vi "多影像平均_二值化_抓邊 - 複製.vi"() -> ()   [LabVIEW 2015]
uses:
  <vilib>/vision/Measure.llb/Edge Options.ctl
  <vilib>/vision/Measure.llb/Edge Polarity.ctl
  <vilib>/userdefined/High Color/IMAQdx.ctl
  <vilib>/Utility/miscctls.llb/LVPositionTypeDef.ctl
  <vilib>/vision/NI_Vision_Development_Module.lvlib
  <vilib>/vision/driver/NI_Vision_Acquisition_Software.lvlib
  <resource>/objmgr/imaqdx.rc
panel:
  in  "載入影像":bool
  in  "拍攝影像":bool
  in  "影像數量":i32=4
  out "二值化影像陣列":T1[](array[plugin-control])
  out "全部影像Histograph":T2(graph)
  out "Image binary":T1(plugin-control)
  out "平均影像Histograph":T3(graph)
  out "Standard Deviation":sgl format="%#.2f"
  out "Mean":sgl format="%#.2f"
  out "影像陣列":T1[](array[plugin-control])
  in  "stop":bool
  in  "Horizontal Progress Bar":u8(slide) scale=0.0..255.0
  out "Image mean":T1(plugin-control)
  out "取像編號":i32
  out "取像視窗":T1(plugin-control)
  in  "Session In":T4="cam1"
  out "degrees":sgl
  in  "單點":bool
  in  "Edge Options":T5={"Edge Polarity"=0, "Kernel Size"=3, "Width"=3, "Minimum Edge Strength"=10.0, "Interpolation Type"=enum."Bilinear Fixed", "Data Processing Method"=enum."Average"} {"Edge Polarity" items=["All Edges", "Rising Edges", "Falling Edges"]; "Minimum Edge Strength" format="%.2f"; "Width" step=2; "Kernel Size" step=2}
  out "Gradient Information":dbl[][](graph)
  out "Line Segment":T7 {"Point 2"."Y" format="%.2f"; "Point 2"."X" format="%.2f"; "Point 1"."Y" format="%.2f"; "Point 1"."X" format="%.2f"}
  out "error out":errorcluster
  in  "Direction":T8(ring)
  in  "Process":u16(ring) items=["Get First Edge", "Get First + Last Edge", "Get All Edges", "Get Best Edge"]
  out "Line Profile":T9(graph)
  in  "Gap":i32=10
  out "Image":T1(plugin-control)
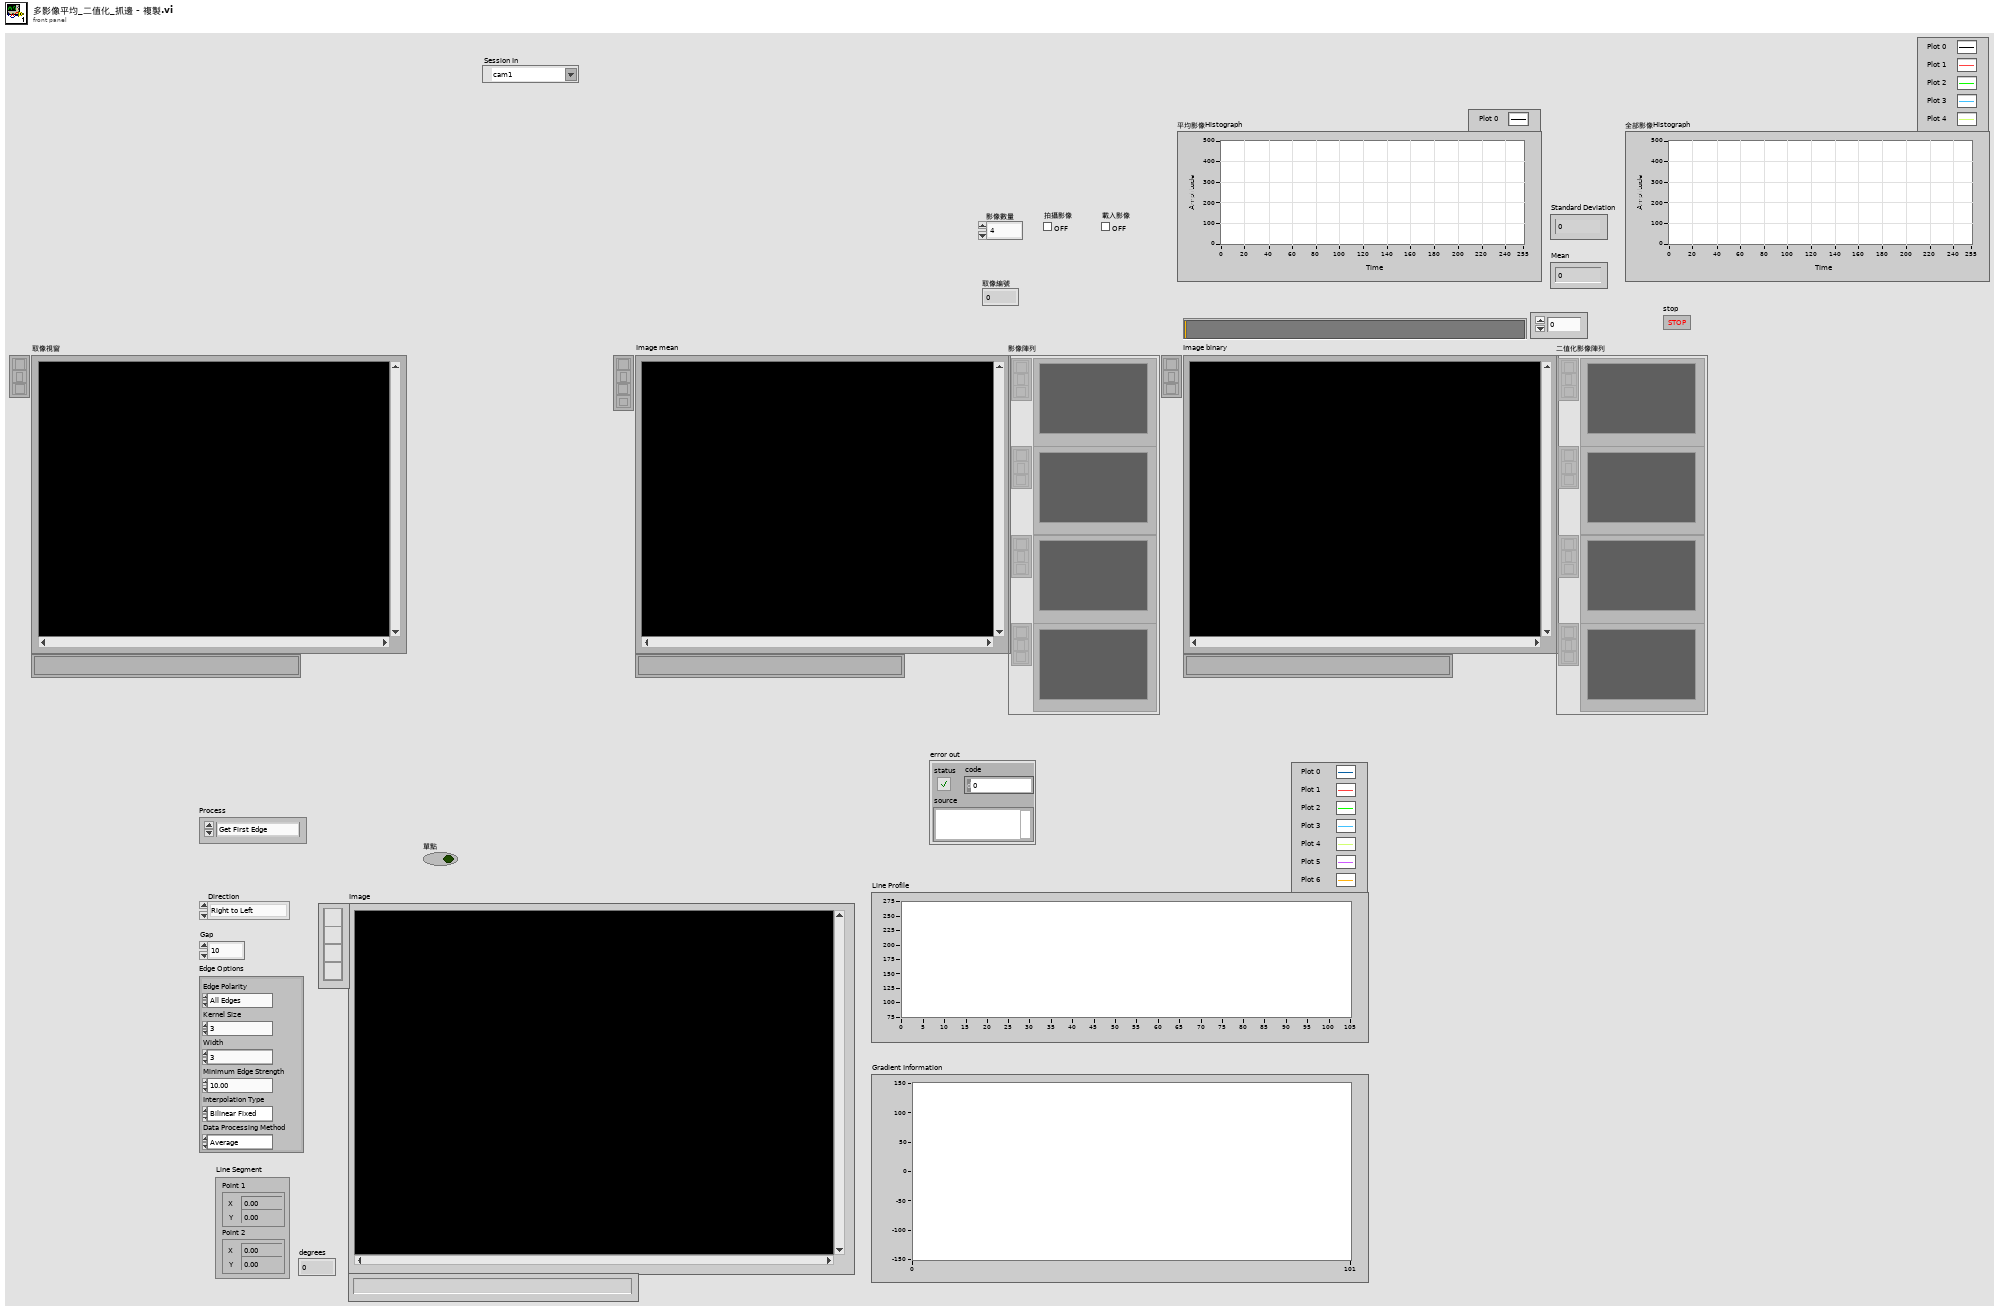
[diagram p1: front panel]
types:
  T1 = typedef "IMAQ Image.ctl" = refnum<image>
  T2 = cluster{"Starting Value":sgl, "Incremental Value":sgl, "Histogram":u32[]}[]
  T3 = cluster{"Starting Value":sgl, "Incremental Value":sgl, "Histogram":u32[]}
  T4 = typedef "IMAQdx.ctl" = refnum<k21>
  T5 = typedef "Edge Options.ctl" = cluster{"Edge Polarity":T6, "Kernel Size":u32, "Width":u32, "Minimum Edge Strength":sgl, "Interpolation Type":enum32{"Zero Order", "Bilinear", "Quadratic", "Cubic", "Bilinear Fixed"}, "Data Processing Method":enum32{"Average", "Median"}}
  T6 = typedef "Edge Polarity.ctl" = u32
  T7 = cluster{"Point 1":cluster{"X":sgl, "Y":sgl}, "Point 2":cluster{"X":sgl, "Y":sgl}}
  T8 = enum16{"Right to Left", "Left  to Right", "Up to Down", "Down to Up"}
  T9 = cluster{"x0":sgl, "dx":sgl, "Pixels Line":sgl[]}[]
  T10 = typedef "LVPositionTypeDef.ctl" = cluster{"Left":i32, "Top":i32}
  T11 = typedef "Image Type" = u32
  T12 = cluster{"Global Rectangle":i32[], "Contours":cluster{"Contour Type":u32, "ROI Type":u32, "Points":i32[]}[]}
  T13 = typedef "IMAQ Rectangle" = cluster{"Left":i32, "Top":i32, "Right":i32, "Bottom":i32, "Rotation":dbl}
  T14 = typedef "IMAQ Line" = cluster{"Start X":i32, "Start Y":i32, "End X":i32, "End Y":i32}
  T15 = typedef "IMAQ Point" = cluster{"X":sgl, "Y":sgl}
  T16 = typedef "ROI Descriptor" = cluster{"Global Rectangle":i32[], "Contours":cluster{"ID":enum32{"External", "Internal"}, "Type":u32, "Coordinates":i32[]}[]}
  T17 = typedef "Edge New.ctl" = cluster{"Location (Pixel)":cluster{"X":sgl, "Y":sgl}, "Location (Real-World)":cluster{"X":sgl, "Y":sgl}, "Distance (Pixel)":dbl, "Distance (Real-World)":dbl, "Strength":dbl, "Noise":dbl, "Rising?":bool}
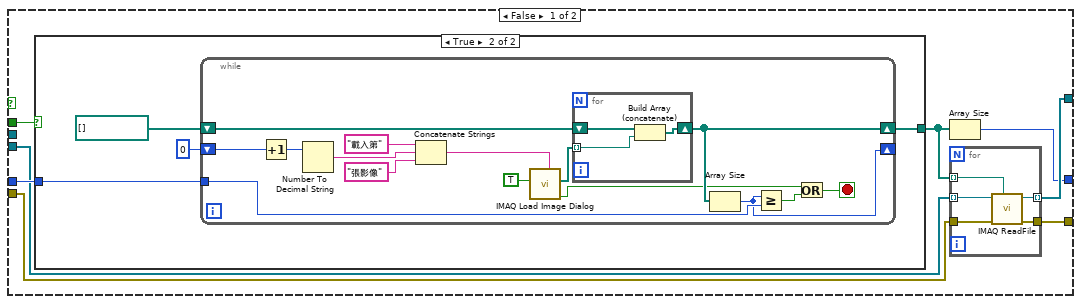
[diagram p2: hidden frame]
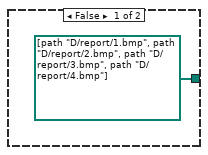
[diagram p3: hidden frame]
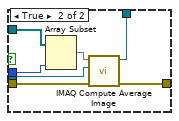
[diagram p4: hidden frame]
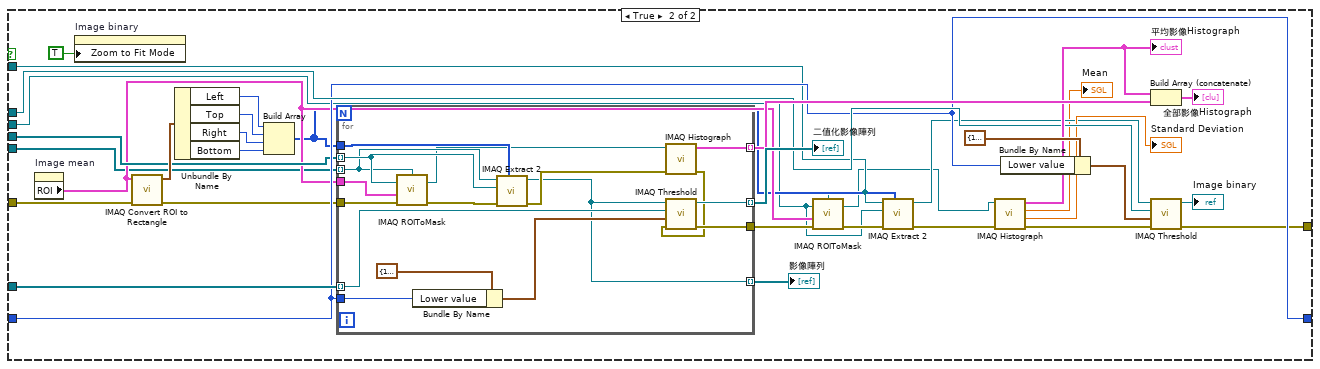
[diagram p5: hidden frame]
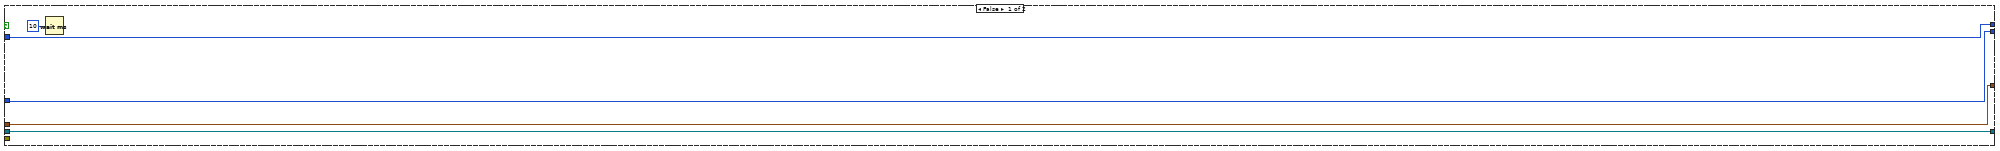
[diagram p6: hidden frame]
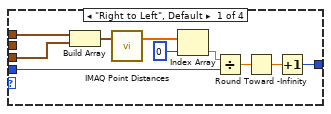
[diagram p7: hidden frame]
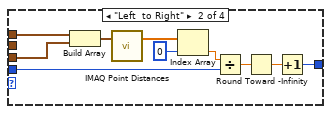
[diagram p8: hidden frame]
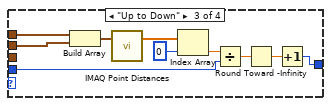
[diagram p9: hidden frame]
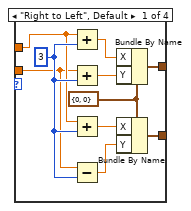
[diagram p12: hidden frame]
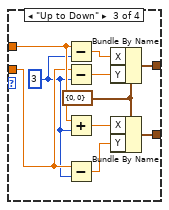
[diagram p13: hidden frame]
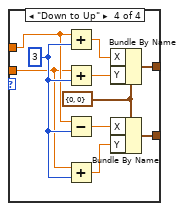
[diagram p14: hidden frame]
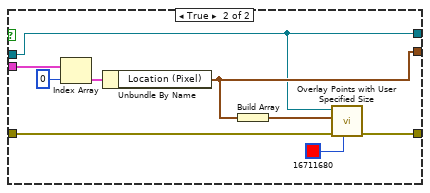
[diagram p15: hidden frame]
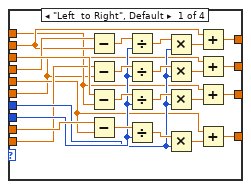
[diagram p16: hidden frame]
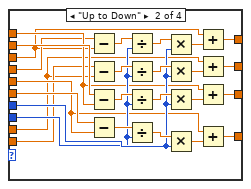
[diagram p17: hidden frame]
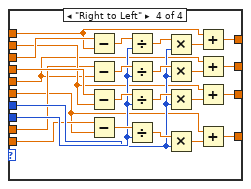
[diagram p18: hidden frame]
diagram:
  w40 = T11 0 items=["Grayscale (U8)", "Grayscale (I16)", "Grayscale (SGL)", "Complex (CSG)", "RGB (U32)", "HSL (U32)", "RGB (U64)", "Grayscale (U16)"] ("Image Type")
  w42 = i32[] [2] items=["No  event", "Click event", "Draw event", "Move event", "Size event", "Scroll event", "Activate event", "Close event", "Double click event"] ("Events list (all)")
  n1 = property on="Pane" class="Pane"("Origin"=T10 {"Left"=-5267, "Top"=-1496} ("Position")) -> (error out=w5:errorcluster)  [unwired: 2 in, 1 out]
  n2 = flat-sequence {
    tunnel: [w68] -> w38
    tunnel: [w67] -> w37
    tunnel: [w65] -> w36
    tunnel: "影像數量" -> [w61]
    tunnel: [w63] -> w35
    tunnel: "拍攝影像" -> [w63]
    tunnel: [w62] -> w34
    tunnel: "載入影像" -> [w62]
    tunnel: [w61] -> w33
    tunnel: [w60] -> w32
    tunnel: [w57] -> w31
    tunnel: [w55] -> w30
    tunnel: [w53] -> w29
    tunnel: [w46] -> w28
    tunnel: w5 -> [w45]
    tunnel: w38 -> [w103]
    tunnel: w37 -> [w104]
    tunnel: [w102] -> w27
    tunnel: w36 -> [w101]
    tunnel: [w101] -> w26
    tunnel: w35 -> [w100]
    tunnel: w34 -> [w99]
    tunnel: w33 -> [w98]
    tunnel: [w97] -> w25
    tunnel: [w96] -> w24
    tunnel: w32 -> [w95]
    tunnel: [w95] -> w23
    tunnel: [w94] -> w22
    tunnel: w31 -> [w94]
    tunnel: w30 -> [w93]
    tunnel: [w93] -> w21
    tunnel: [w92] -> w20
    tunnel: w29 -> [w92]
    tunnel: w28 -> [w91]
    tunnel: w27 -> [w165]
    tunnel: w26 -> [w171]
    tunnel: w25 -> [w170]
    tunnel: w24 -> [w162]
    tunnel: w23 -> [w169]
    tunnel: [w169] -> w19
    tunnel: [w166] -> w18
    tunnel: [w165] -> w17
    tunnel: [w164] -> w16
    tunnel: [w168] -> w15
    tunnel: w22 -> [w168]
    tunnel: w21 -> [w163]
    tunnel: [w163] -> w14
    tunnel: [w167] -> w13
    tunnel: w20 -> [w167]
    tunnel: w19 -> [w191]
    tunnel: w18 -> [w186]
    tunnel: w17 -> [w192]
    tunnel: w16 -> [w184]
    tunnel: w15 -> [w190]
    tunnel: w14 -> [w185]
    tunnel: w13 -> [w187]
    tunnel: [w184] -> w9
    tunnel: [w183] -> w4
    frame #0 {
      w59 = T11 0 items=["Grayscale (U8)", "Grayscale (I16)", "Grayscale (SGL)", "Complex (CSG)", "RGB (U32)", "HSL (U32)", "RGB (U64)", "Grayscale (U16)"] ("Image Type")
      w52 = 20
      w64 = T11 0 items=["Grayscale (U8)", "Grayscale (I16)", "Grayscale (SGL)", "Complex (CSG)", "RGB (U32)", "HSL (U32)", "RGB (U64)", "Grayscale (U16)"] ("Image Type")
      n3 = call <vilib>:"IMAQdx Open Camera.vi"("error in"=w45, "Session In"="Session In") -> ("error out"=w54:errorcluster, "Session Out"=w68:T4)  [unwired: 8 in]
      n4 = for {
        N: w52 -> [_]
        tunnel: [w90] -> w67 mode=indexing
        tunnel: w54 -> [w89]
        tunnel: [w88] -> w51
        i -> [w87]
        n5 = Number To Decimal String(number=w87) -> (decimal integer string=w85:string)  [unwired: 1 in]
        n6 = Concatenate Strings("Image", w85) -> (w84:string)
        n7 = call "IMAQ Create"("Image Name"=w84, "error in (no error)"=w89) -> ("New Image"=w90:T1, "error out"=w88:errorcluster)  [unwired: 3 in]
      }
      n8 = for {
        N: w52 -> [_]
        tunnel: [w76] -> w53 mode=indexing
        tunnel: w51 -> [w75]
        tunnel: [w70] -> _
        tunnel: [w70] -> w50 mode=indexing
        i -> [w74]
        n9 = Number To Decimal String(number=w74) -> (decimal integer string=w72:string)  [unwired: 1 in]
        n10 = Concatenate Strings("Histogram Mask", w72) -> (w71:string)
        n11 = call "IMAQ Create"("Image Name"=w71, "error in (no error)"=w75) -> ("New Image"=w76:T1, "error out"=w70:errorcluster)  [unwired: 3 in]
      }
      n12 = for {
        N: w52 -> [_]
        tunnel: [w83] -> w60 mode=indexing
        tunnel: w50 -> [w82] mode=indexing
        tunnel: [w81] -> w47
        i -> [w80]
        n13 = Number To Decimal String(number=w80) -> (decimal integer string=w78:string)  [unwired: 1 in]
        n14 = Concatenate Strings("Threshole", w78) -> (w77:string)
        n15 = call "IMAQ Create"("Image Name"=w77, "error in (no error)"=w82) -> ("New Image"=w83:T1, "error out"=w81:errorcluster)  [unwired: 3 in]
      }
      n16 = call "IMAQ Create"("Image Name"="imageMeans", "Image Type"=w64, "error in (no error)"=w47) -> ("New Image"=w65:T1, "error out"=w49:errorcluster)  [unwired: 2 in]
      n17 = call "IMAQ Create"("Image Name"="Histogram Mask", "error in (no error)"=w49) -> ("New Image"=w55:T1, "error out"=w48:errorcluster)  [unwired: 3 in]
      n18 = call "IMAQ Create"("Image Name"="imageBinary", "Image Type"=w59, "error in (no error)"=w48) -> ("New Image"=w57:T1, "error out"=w46:errorcluster)  [unwired: 2 in]
    }
    frame #1 {
      n19 = case shown="True" w100 {
        tunnel: w104 -> [w109 w147]
        tunnel: w103 -> [_ w146]
        tunnel: w91 -> [w108 w144]
        tunnel: [w110 w143] -> w102
        tunnel: w99 -> [w112 _]
        tunnel: w98 -> [w111 w141]
        tunnel: [w107 w142] -> w97
        tunnel: [w105 w141] -> w96
        frame False {
          n20 = case shown="True" w112 {
            tunnel: [path[] [path "D:/report/1.bmp", path "D:/report/2.bmp", path "D:/report/3.bmp", path "D:/report/4.bmp"] w117] -> w106
            tunnel: w111 -> [_ w116]
            frame False {
            }
            frame True {
              n21 = while {
                tunnel: w116 -> [w129]
                shift-right: [w132] -> w117
                shift-left: path[] [] -> [w128]
                shift-right: [w127] -> _
                shift-left: 0 -> [w126]
                stop <- w119 stop-if-true
                n22 = Increment(x=w126) -> (x+1=w125:i32)
                n23 = Number To Decimal String(number=w125) -> (decimal integer string=w122:string)  [unwired: 1 in]
                n24 = Concatenate Strings("載入第", w122, "張影像") -> (w121:string)
                n25 = call "IMAQ Load Image Dialog"("Button Label"=w121, "Multiple Files? (No)"=TRUE) -> ("Cancelled?"=w120:bool, "Paths"=w130:path[])  [unwired: 7 in, 1 out]
                n26 = for {
                  tunnel: w130 -> [w134] mode=indexing
                  shift-right: [w133] -> w132
                  shift-left: w128 -> [w135]
                  n27 = Build Array (concatenate)(w135, w134) -> (w133:path[])
                }
                n28 = Array Size(array=w132) -> (size(s)=w127:i32)
                n29 = Greater Or Equal?(x=w127, y=w129) -> (x >= y?=w118:bool)
                n30 = Or(x=w120, y=w118) -> (x .or. y?=w119:bool)
              }
            }
          }
          n31 = Array Size(array=w106) -> (size(s)=w105:i32)
          n32 = for {
            tunnel: w106 -> [w140] mode=indexing
            tunnel: [w139] -> w110 mode=indexing
            tunnel: w109 -> [w138] mode=indexing
            tunnel: w108 -> [w137]
            tunnel: [w136] -> w107
            n33 = call "IMAQ ReadFile"("File Path"=w140, "error in (no error)"=w137, "Image"=w138) -> ("error out"=w136:errorcluster, "Image Out"=w139:T1)  [unwired: 4 in, 3 out]
          }
        }
        frame True {
          n34 = for {
            N: w141 -> [_]
            tunnel: w147 -> [w148] mode=indexing
            tunnel: w146 -> [w158]
            tunnel: dbl[] [0.01, 0.03, 0.05, 0.07] -> [w157] mode=indexing
            tunnel: w144 -> [w152]
            tunnel: [w156] -> w143 mode=indexing
            tunnel: [w154] -> w142
            i -> [w159]
            w155 = T11 0 items=["Grayscale (U8)", "Grayscale (I16)", "Grayscale (SGL)", "Complex (CSG)", "RGB (U32)", "HSL (U32)", "RGB (U64)", "Grayscale (U16)"] ("Image Type")
            n35 = property class="IMAQdx"(reference=w158, error in=w152, "ActiveAttribute"="CameraAttributes::Exposure::Value", "ValueDBL"=w157) -> (reference out=w149:T4, error out=w151:errorcluster)
            n36 = call <vilib>:"IMAQdx Snap2.vi"("error in"=w151, "Image In"=w148, "Session In"=w149) -> ("error out"=w154:errorcluster, "Image Out"=w153:T1)  [unwired: 6 in, 1 out]
            "取像視窗" <- w153
            n37 = call "IMAQ Cast Image"("Image Type"=w155, "Image Src"=w153) -> ("Image Dst Out"=w156:T1)  [unwired: 8 in, 1 out]
            "取像編號" <- w159
          }
        }
      }
    }
    frame #2 {
      n38 = Not Equal?(x=w162, y=1) -> (x != y?=w160:bool)
      n39 = case shown="False" w160 {
        tunnel: w171 -> [_ w182]
        tunnel: w170 -> [w175 w181]
        tunnel: w162 -> [_ w180]
        tunnel: [w175 w178] -> w166
        tunnel: w165 -> [w173 w177]
        tunnel: [w172 w176] -> w164
        frame False {
          n40 = Index Array(array=w173, index=0) -> (element=w172:T1)
        }
        frame True {
          n41 = Array Subset(array=w177, length=w180) -> (w179:T1[])  [unwired: 1 in]
          n42 = call "IMAQ Compute Average Image"("error in (no error)"=w181, "Image Dst"=w182, "Images"=w179) -> ("error out"=w178:errorcluster, "Image Dst Out"=w176:T1)  [unwired: 7 in]
        }
      }
      "Image mean" <- w164
    }
    frame #3 {
      w188 = i32[] [2] items=["No  event", "Click event", "Draw event", "Move event", "Size event", "Scroll event", "Activate event", "Close event", "Double click event"] ("Events list (all)")
      n43 = property on="Image mean" class="ImageControl"("ROI"=T12 {"Global Rectangle"=[0, 0, 1292, 964], "Contours"=[{"Contour Type"=0, "ROI Type"=3, "Points"=[0, 0, 1292, 964]}]}) -> ()  [unwired: 2 in, 2 out]
      n44 = while {
        tunnel: w192 -> [w212]
        tunnel: w191 -> [w211]
        tunnel: w184 -> [w209]
        tunnel: w185 -> [w210]
        tunnel: w190 -> [w208]
        tunnel: w188 -> [w206]
        shift-right: [w203] -> _
        shift-left: _ -> [w201]
        tunnel: w187 -> [w196]
        tunnel: w186 -> [w195]
        tunnel: [w193] -> w183
        i -> [w204]
        stop <- "stop" stop-if-true
        n45 = invoke on="Image mean" class="ImageControl" method="Get Last Event"("Which Events"=w206) -> ("Type"=w205:i32)  [unwired: 7 in, 7 out]
        n46 = Not Equal To 0?(x=w205) -> (x != 0?=w199:bool)
        n47 = Not Equal?(x="Horizontal Progress Bar", y=w201) -> (x != y?=w198:bool)
        n48 = Equal To 0?(x=w204) -> (x = 0?=w200:bool)
        n49 = Compound Arithmetic op=OR(w200, w199, w198) -> (w197:bool)
        n50 = case shown="False" w197 {
          tunnel: w212 -> [_ w221]
          tunnel: w211 -> [_ w249]
          tunnel: w210 -> [_ w218]
          tunnel: w209 -> [_ w219]
          tunnel: w208 -> [_ w236]
          tunnel: "Horizontal Progress Bar" -> [w214 w234]
          tunnel: [w214 w234] -> w203
          tunnel: w196 -> [_ w232]
          tunnel: w195 -> [w213 w223]
          tunnel: [w213 w216] -> w193
          frame False {
            n51 = Wait (ms)(milliseconds to wait=u32 10) -> ()  [unwired: 1 out]
          }
          frame True {
            n52 = property on="Image mean" class="ImageControl"() -> ("ROI"=w231:T12)  [unwired: 2 in, 2 out]
            n53 = property on="Image binary" class="ImageControl"("Zoom to Fit Mode"=TRUE) -> ()  [unwired: 2 in, 2 out]
            n54 = call "IMAQ Convert ROI to Rectangle"("error in (no error)"=w223, "ROI Descriptor"=w231) -> ("error out"=w224:errorcluster, "Rectangle"=w241:T13)  [unwired: 7 in]
            n55 = Unbundle By Name(w241) -> ("Left"=w237:i32, "Top"=w238:i32, "Right"=w239:i32, "Bottom"=w240:i32)
            n56 = Build Array(w237, w238, w239, w240) -> (w230:i32[])
            n57 = for {
              tunnel: w221 -> [w252] mode=indexing
              tunnel: w249 -> [w266] mode=indexing
              tunnel: [w265] -> w248 mode=indexing
              tunnel: [w253] -> w244 mode=indexing
              tunnel: w234 -> [w262]
              tunnel: w232 -> [w259] mode=indexing
              tunnel: w231 -> [w261]
              tunnel: w230 -> [w260]
              tunnel: [w256] -> w225
              tunnel: w224 -> [w255]
              tunnel: [w254] -> w220 mode=indexing
              n58 = call "IMAQ ROIToMask"("error in (no error)"=w255, "ROI Descriptor"=w261, "Image"=w259, "Image Model"=w252) -> ("error out"=w258:errorcluster, "Image Out"=w251:T1)  [unwired: 2 in, 1 out]
              n59 = Bundle By Name(cluster=cluster{"Lower value":sgl, "Upper value":sgl} {"Lower value"=128.0, "Upper value"=255.0} ("Range"), "Lower value"=w262) -> (w263:cluster{"Lower value":sgl, "Upper value":sgl})
              n60 = call "IMAQ Extract 2"("Optional Rectangle"=w260, "error in (no error)"=w258, "Image Dst"=w259, "Image Src"=w252) -> ("error out"=w257:errorcluster, "Image Dst Out"=w254:T1)  [unwired: 6 in]
              n61 = call "IMAQ Histograph"("error in (no error)"=w257, "Image"=w251) -> ("error out"=w250:errorcluster, "Histogram Graph"=w253:T3)  [unwired: 6 in, 2 out]
              n62 = call "IMAQ Threshold"("error in (no error)"=w250, "Range"=w263, "Image Dst"=w266, "Image Src"=w254) -> ("error out"=w256:errorcluster, "Image Dst Out"=w265:T1)  [unwired: 6 in]
            }
            "二值化影像陣列" <- w248
            "影像陣列" <- w220
            n63 = call "IMAQ ROIToMask"("error in (no error)"=w225, "ROI Descriptor"=w231, "Image"=w218, "Image Model"=w219) -> ("error out"=w228:errorcluster, "Image Out"=w217:T1)  [unwired: 2 in, 1 out]
            n64 = call "IMAQ Extract 2"("Optional Rectangle"=w230, "error in (no error)"=w228, "Image Dst"=w218, "Image Src"=w219) -> ("error out"=w227:errorcluster, "Image Dst Out"=w229:T1)  [unwired: 6 in]
            n65 = call "IMAQ Histograph"("error in (no error)"=w227, "Image"=w217) -> ("error out"=w226:errorcluster, "Standard  Deviation"=→"Standard Deviation":sgl, "Mean Value"=→"Mean":sgl, "Histogram Graph"=w242:T3)  [unwired: 6 in]
            "平均影像Histograph" <- w242
            n66 = Bundle By Name(cluster=cluster{"Lower value":sgl, "Upper value":sgl} {"Lower value"=128.0, "Upper value"=255.0} ("Range"), "Lower value"=w234) -> (w247:cluster{"Lower value":sgl, "Upper value":sgl})
            n67 = Build Array (concatenate)(w242, w244) -> (→"全部影像Histograph":T2)
            n68 = call "IMAQ Threshold"("error in (no error)"=w226, "Range"=w247, "Image Dst"=w236, "Image Src"=w229) -> ("error out"=w216:errorcluster, "Image Dst Out"=→"Image binary":T1)  [unwired: 6 in]
          }
        }
        n69 = property on="平均影像Histograph" class="WFGraph (strict)"() -> ("YScale.Maximum"=w194:dbl)  [unwired: 2 in, 2 out]
        n70 = property on="全部影像Histograph" class="WFGraph (strict)"("YScale.Maximum"=w194) -> ()  [unwired: 2 in, 2 out]
      }
    }
  }
  n71 = property on="Image" class="ImageControl"("ROI"=T12 {"Global Rectangle"=[450, 180, 600, 400], "Contours"=[{"Contour Type"=0, "ROI Type"=3, "Points"=[450, 180, 600, 400]}]}) -> ()  [unwired: 2 in, 2 out]
  n72 = property on="Pane" class="Pane"(error in=w4, "Origin"=T10 {"Left"=-5844, "Top"=-513} ("Position")) -> (error out=w3:errorcluster)  [unwired: 1 in, 1 out]
  n73 = call "IMAQ Create"("Image Name"="Edge Detection Source", "error in (no error)"=w3) -> ("New Image"=w7:T1, "error out"=w6:errorcluster)  [unwired: 3 in]
  n74 = call "IMAQ Copy"("Image Dst"=w7, "Image Src"=w9) -> ("Image Dst Out"=w8:T1)  [unwired: 4 in, 1 out]
  n75 = call "IMAQ Cast Image"("Image Type"=w40, "error in (no error)"=w6, "Image Src"=w8) -> ("error out"=w39:errorcluster, "Image Dst Out"=w41:T1)  [unwired: 7 in]
  n76 = while {
    tunnel: w39 -> [w284]
    tunnel: w41 -> [w285]
    tunnel: w42 -> [w283]
    shift-right: [w281] -> _
    shift-left: _ -> [w280]
    shift-right: [w273] -> _
    shift-left: _ -> [w274]
    shift-right: [w268] -> _
    shift-left: _ -> [w269]
    stop <- FALSE stop-if-true
    n77 = invoke on="Image" class="ImageControl" method="Get Last Event"("Which Events"=w283) -> ("Type"=w282:i32)  [unwired: 7 in, 7 out]
    n78 = Not Equal?(x=w280, y="Direction") -> (x != y?=w279:bool)
    n79 = Not Equal To 0?(x=w282) -> (x != 0?=w278:bool)
    n80 = Not Equal?(x=w274, y="Gap") -> (x != y?=w272:bool)
    n81 = Not Equal?(x=w269, y="Edge Options") -> (x != y?=w267:bool)
    n82 = Compound Arithmetic op=OR(w279, w278, w272, w267) -> (w277:bool)
    n83 = case shown="True" w277 {
      tunnel: w285 -> [w288 w344]
      tunnel: w284 -> [_ w343]
      tunnel: "Direction" -> [w290 w334]
      tunnel: [w290 w334] -> w281
      tunnel: "Gap" -> [w289 w333]
      tunnel: [w289 w333] -> w273
      tunnel: [w288 w304] -> w271
      tunnel: "Edge Options" -> [w287 w313]
      tunnel: [w287 w313] -> w268
      frame False {
        n84 = Wait (ms)(milliseconds to wait=u32 10) -> ()  [unwired: 1 out]
      }
      frame True {
        n85 = call "IMAQ Clear Overlay"("error in (no error)"=w343, "Image"=w344) -> ("error out"=w342:errorcluster, "Image Out"=w316:T1)  [unwired: 8 in]
        n86 = property on="Image" class="ImageControl"() -> ("ROI"=w345:T12)  [unwired: 2 in, 2 out]
        n87 = call "IMAQ Convert ROI to Rectangle"("error in (no error)"=w342, "ROI Descriptor"=w345) -> ("error out"=w315:errorcluster, "Rectangle"=w337:T13)  [unwired: 7 in]
        n88 = call "IMAQ Convert Rectangle to ROI (Polygon)"("Rectangle"=w337) -> ("Rectangle Points"=w330:T15[])  [unwired: 7 in, 2 out]
        n89 = Index Array(array=w330, index #1=0 ("index"), index #2=1 ("index"), index #3=2 ("index"), index #4=3 ("index")) -> (element #1=w332:T15, element #2=w331:T15, element #3=w322:T15, element #4=w323:T15)
        n90 = case shown="\"Down to Up\"" w334 {
          tunnel: w333 -> [w353 w363 w373 w383]
          tunnel: [w352 w362 w372 w382] -> w329
          tunnel: w332 -> [w349 w359 w371 w379]
          tunnel: w323 -> [w348 w358 _ _]
          tunnel: w331 -> [_ _ w367 w378]
          frame "Right to Left", Default {
            n91 = Build Array(w349, w348) -> (w351:T15[])
            n92 = call "IMAQ Point Distances"("Points"=w351) -> ("Distances"=w350:sgl[])  [unwired: 4 in, 1 out]
            n93 = Index Array(array=w350, index=0) -> (element=w346:sgl)
            n94 = Divide(x=w346, y=w353) -> (x/y=w354:sgl)
            n95 = Round Toward -Infinity(1:w354) -> (0:w355:sgl)
            n96 = Increment(x=w355) -> (x+1=w352:i32)
          }
          frame "Left  to Right" {
            n97 = Build Array(w359, w358) -> (w361:T15[])
            n98 = call "IMAQ Point Distances"("Points"=w361) -> ("Distances"=w360:sgl[])  [unwired: 4 in, 1 out]
            n99 = Index Array(array=w360, index=0) -> (element=w356:sgl)
            n100 = Divide(x=w356, y=w363) -> (x/y=w364:sgl)
            n101 = Round Toward -Infinity(1:w364) -> (0:w365:sgl)
            n102 = Increment(x=w365) -> (x+1=w362:i32)
          }
          frame "Up to Down" {
            n103 = Build Array(w371, w367) -> (w370:T15[])
            n104 = call "IMAQ Point Distances"("Points"=w370) -> ("Distances"=w369:sgl[])  [unwired: 4 in, 1 out]
            n105 = Index Array(array=w369, index=0) -> (element=w368:sgl)
            n106 = Divide(x=w368, y=w373) -> (x/y=w374:sgl)
            n107 = Round Toward -Infinity(1:w374) -> (0:w375:sgl)
            n108 = Increment(x=w375) -> (x+1=w372:i32)
          }
          frame "Down to Up" {
            n109 = Build Array(w379, w378) -> (w381:T15[])
            n110 = call "IMAQ Point Distances"("Points"=w381) -> ("Distances"=w380:sgl[])  [unwired: 4 in, 1 out]
            n111 = Index Array(array=w380, index=0) -> (element=w377:sgl)
            n112 = Divide(x=w377, y=w383) -> (x/y=w384:sgl)
            n113 = Round Toward -Infinity(1:w384) -> (0:w385:sgl)
            n114 = Increment(x=w385) -> (x+1=w382:i32)
          }
        }
        n115 = Unbundle By Name(w332) -> ("X"=w327:sgl, "Y"=w326:sgl)
        n116 = Unbundle By Name(w331) -> ("X"=w320:sgl, "Y"=w318:sgl)
        n117 = Unbundle By Name(w323) -> ("X"=w328:sgl, "Y"=w317:sgl)
        n118 = Unbundle By Name(w322) -> ("X"=w321:sgl, "Y"=w319:sgl)
        n119 = for {
          N: w329 -> [w415]
          tunnel: w334 -> [w406]
          tunnel: w328 -> [w445]
          tunnel: w327 -> [w444]
          tunnel: w317 -> [w443]
          tunnel: w326 -> [w442]
          tunnel: w321 -> [w441]
          tunnel: w320 -> [w440]
          tunnel: w319 -> [w439]
          tunnel: w318 -> [w438]
          tunnel: [w427] -> w309
          tunnel: w316 -> [w410]
          tunnel: w315 -> [w436]
          tunnel: [w425] -> w308
          tunnel: "Process" -> [w428]
          tunnel: w313 -> [w424]
          tunnel: [w422] -> w312 mode=indexing
          tunnel: [w421] -> w311 mode=indexing
          tunnel: [w420] -> w310 mode=indexing
          i -> [w416]
          w414 = 1
          w408 = u32 16860 ("Color")
          w404 = cluster{"X":i32, "Y":i32} {"X"=0, "Y"=0} ("Start Point")
          n120 = Equal?(x=w416, y=w414) -> (x = y?=w412:bool)
          n121 = Subtract(x=w415, y=w414) -> (x-y=w413:i32)
          n122 = case shown="\"Down to Up\"" w406 {
            tunnel: [w529 w548 w574 w599] -> w435
            tunnel: [w524 w547 w573 w600] -> w403
            tunnel: [w527 w545 w571 w597] -> w434
            tunnel: [w523 w546 w572 w598] -> w405
            tunnel: w445 -> [w542 w553 w579 w609]
            tunnel: w444 -> [w520 w555 w578 w608]
            tunnel: w415 -> [w533 w557 w584 w610]
            tunnel: w416 -> [w532 w558 w575 w607]
            tunnel: w443 -> [w539 w549 w581 w604]
            tunnel: w442 -> [w522 w551 w580 w603]
            tunnel: w441 -> [w536 w554 w577 w606]
            tunnel: w440 -> [w521 w556 w576 w605]
            tunnel: w439 -> [w531 w550 w582 w602]
            tunnel: w438 -> [w519 w552 w583 w601]
            frame "Left  to Right", Default {
              n123 = Subtract(x=w536, y=w521) -> (x-y=w538:sgl)
              n124 = Subtract(x=w531, y=w519) -> (x-y=w534:sgl)
              n125 = Subtract(x=w542, y=w520) -> (x-y=w543:sgl)
              n126 = Subtract(x=w539, y=w522) -> (x-y=w541:sgl)
              n127 = Divide(x=w538, y=w533) -> (x/y=w537:sgl)
              n128 = Divide(x=w534, y=w533) -> (x/y=w535:sgl)
              n129 = Divide(x=w543, y=w533) -> (x/y=w544:sgl)
              n130 = Divide(x=w541, y=w533) -> (x/y=w540:sgl)
              n131 = Multiply(x=w537, y=w532) -> (x*y=w526:sgl)
              n132 = Multiply(x=w535, y=w532) -> (x*y=w525:sgl)
              n133 = Multiply(x=w544, y=w532) -> (x*y=w530:sgl)
              n134 = Multiply(x=w540, y=w532) -> (x*y=w528:sgl)
              n135 = Add(x=w521, y=w526) -> (x+y=w524:sgl)
              n136 = Add(x=w519, y=w525) -> (x+y=w523:sgl)
              n137 = Add(x=w520, y=w530) -> (x+y=w529:sgl)
              n138 = Add(x=w522, y=w528) -> (x+y=w527:sgl)
            }
            frame "Up to Down" {
              n139 = Subtract(x=w554, y=w553) -> (x-y=w566:sgl)
              n140 = Subtract(x=w550, y=w549) -> (x-y=w563:sgl)
              n141 = Subtract(x=w556, y=w555) -> (x-y=w569:sgl)
              n142 = Subtract(x=w552, y=w551) -> (x-y=w568:sgl)
              n143 = Divide(x=w566, y=w557) -> (x/y=w565:sgl)
              n144 = Divide(x=w563, y=w557) -> (x/y=w564:sgl)
              n145 = Divide(x=w569, y=w557) -> (x/y=w570:sgl)
              n146 = Divide(x=w568, y=w557) -> (x/y=w567:sgl)
              n147 = Multiply(x=w565, y=w558) -> (x*y=w560:sgl)
              n148 = Multiply(x=w564, y=w558) -> (x*y=w559:sgl)
              n149 = Multiply(x=w570, y=w558) -> (x*y=w562:sgl)
              n150 = Multiply(x=w567, y=w558) -> (x*y=w561:sgl)
              n151 = Add(x=w553, y=w560) -> (x+y=w547:sgl)
              n152 = Add(x=w549, y=w559) -> (x+y=w546:sgl)
              n153 = Add(x=w555, y=w562) -> (x+y=w548:sgl)
              n154 = Add(x=w551, y=w561) -> (x+y=w545:sgl)
            }
            frame "Down to Up" {
              n155 = Subtract(x=w576, y=w578) -> (x-y=w595:sgl)
              n156 = Subtract(x=w583, y=w580) -> (x-y=w594:sgl)
              n157 = Subtract(x=w577, y=w579) -> (x-y=w592:sgl)
              n158 = Subtract(x=w582, y=w581) -> (x-y=w589:sgl)
              n159 = Divide(x=w595, y=w584) -> (x/y=w596:sgl)
              n160 = Divide(x=w594, y=w584) -> (x/y=w593:sgl)
              n161 = Divide(x=w592, y=w584) -> (x/y=w591:sgl)
              n162 = Divide(x=w589, y=w584) -> (x/y=w590:sgl)
              n163 = Multiply(x=w596, y=w575) -> (x*y=w588:sgl)
              n164 = Multiply(x=w593, y=w575) -> (x*y=w587:sgl)
              n165 = Multiply(x=w591, y=w575) -> (x*y=w586:sgl)
              n166 = Multiply(x=w590, y=w575) -> (x*y=w585:sgl)
              n167 = Add(x=w578, y=w588) -> (x+y=w573:sgl)
              n168 = Add(x=w580, y=w587) -> (x+y=w572:sgl)
              n169 = Add(x=w579, y=w586) -> (x+y=w574:sgl)
              n170 = Add(x=w581, y=w585) -> (x+y=w571:sgl)
            }
            frame "Right to Left" {
              n171 = Subtract(x=w609, y=w608) -> (x-y=w621:sgl)
              n172 = Subtract(x=w604, y=w603) -> (x-y=w620:sgl)
              n173 = Subtract(x=w606, y=w605) -> (x-y=w618:sgl)
              n174 = Subtract(x=w602, y=w601) -> (x-y=w615:sgl)
              n175 = Divide(x=w621, y=w610) -> (x/y=w622:sgl)
              n176 = Divide(x=w620, y=w610) -> (x/y=w619:sgl)
              n177 = Divide(x=w618, y=w610) -> (x/y=w617:sgl)
              n178 = Divide(x=w615, y=w610) -> (x/y=w616:sgl)
              n179 = Multiply(x=w622, y=w607) -> (x*y=w614:sgl)
              n180 = Multiply(x=w619, y=w607) -> (x*y=w613:sgl)
              n181 = Multiply(x=w617, y=w607) -> (x*y=w612:sgl)
              n182 = Multiply(x=w616, y=w607) -> (x*y=w611:sgl)
              n183 = Add(x=w608, y=w614) -> (x+y=w600:sgl)
              n184 = Add(x=w603, y=w613) -> (x+y=w598:sgl)
              n185 = Add(x=w605, y=w612) -> (x+y=w599:sgl)
              n186 = Add(x=w601, y=w611) -> (x+y=w597:sgl)
            }
          }
          n187 = Equal?(x=w416, y=w413) -> (x = y?=w411:bool)
          n188 = Or(x=w412, y=w411) -> (x .or. y?=w401:bool)
          n189 = Bundle By Name(cluster=w404, "X"=w403, "Y"=w405) -> (w402:cluster{"X":i32, "Y":i32})
          n190 = Bundle By Name(cluster=w404, "X"=w435, "Y"=w434) -> (w437:cluster{"X":i32, "Y":i32})
          n191 = Bundle By Name(cluster=T14 {"Start X"=0, "Start Y"=0, "End X"=0, "End Y"=0} ("Line"), "Start X"=w435, "Start Y"=w434, "End X"=w403, "End Y"=w405) -> (w423:T14)
          n192 = case shown="True" w401 {
            tunnel: w410 -> [w447 w457]
            tunnel: [w447 w456] -> w409
            tunnel: w408 -> [_ w455]
            tunnel: w406 -> [_ w454]
            tunnel: w403 -> [_ w448]
            tunnel: w405 -> [_ w453]
            tunnel: w402 -> [_ w449]
            frame False {
            }
            frame True {
              n193 = case shown="\"Left  to Right\"" w454 {
                tunnel: w448 -> [w459 w471 w483 w491]
                tunnel: w453 -> [w458 w470 w482 w490]
                tunnel: [w461 w469 w480 w489] -> w452
                tunnel: [w460 w468 w479 w488] -> w451
                frame "Right to Left", Default {
                  w463 = cluster{"X":i32, "Y":i32} {"X"=0, "Y"=0} ("Start Point")
                  w462 = 3
                  n194 = Add(x=w459, y=w462) -> (x+y=w464:sgl)
                  n195 = Add(x=w458, y=w462) -> (x+y=w465:sgl)
                  n196 = Add(x=w459, y=w462) -> (x+y=w466:sgl)
                  n197 = Subtract(x=w458, y=w462) -> (x-y=w467:sgl)
                  n198 = Bundle By Name(cluster=w463, "X"=w464, "Y"=w465) -> (w461:cluster{"X":i32, "Y":i32})
                  n199 = Bundle By Name(cluster=w463, "X"=w466, "Y"=w467) -> (w460:cluster{"X":i32, "Y":i32})
                }
                frame "Left  to Right" {
                  w473 = cluster{"X":i32, "Y":i32} {"X"=0, "Y"=0} ("Start Point")
                  w472 = 3
                  n200 = Subtract(x=w471, y=w472) -> (x-y=w474:sgl)
                  n201 = Add(x=w470, y=w472) -> (x+y=w475:sgl)
                  n202 = Subtract(x=w471, y=w472) -> (x-y=w476:sgl)
                  n203 = Subtract(x=w470, y=w472) -> (x-y=w477:sgl)
                  n204 = Bundle By Name(cluster=w473, "X"=w474, "Y"=w475) -> (w469:cluster{"X":i32, "Y":i32})
                  n205 = Bundle By Name(cluster=w473, "X"=w476, "Y"=w477) -> (w468:cluster{"X":i32, "Y":i32})
                }
                frame "Up to Down" {
                  w481 = cluster{"X":i32, "Y":i32} {"X"=0, "Y"=0} ("Start Point")
                  w478 = 3
                  n206 = Subtract(x=w483, y=w478) -> (x-y=w484:sgl)
                  n207 = Subtract(x=w482, y=w478) -> (x-y=w485:sgl)
                  n208 = Add(x=w483, y=w478) -> (x+y=w486:sgl)
                  n209 = Subtract(x=w482, y=w478) -> (x-y=w487:sgl)
                  n210 = Bundle By Name(cluster=w481, "X"=w484, "Y"=w485) -> (w480:cluster{"X":i32, "Y":i32})
                  n211 = Bundle By Name(cluster=w481, "X"=w486, "Y"=w487) -> (w479:cluster{"X":i32, "Y":i32})
                }
                frame "Down to Up" {
                  w493 = cluster{"X":i32, "Y":i32} {"X"=0, "Y"=0} ("Start Point")
                  w492 = 3
                  n212 = Add(x=w491, y=w492) -> (x+y=w494:sgl)
                  n213 = Add(x=w490, y=w492) -> (x+y=w495:sgl)
                  n214 = Subtract(x=w491, y=w492) -> (x-y=w496:sgl)
                  n215 = Add(x=w490, y=w492) -> (x+y=w497:sgl)
                  n216 = Bundle By Name(cluster=w493, "X"=w494, "Y"=w495) -> (w489:cluster{"X":i32, "Y":i32})
                  n217 = Bundle By Name(cluster=w493, "X"=w496, "Y"=w497) -> (w488:cluster{"X":i32, "Y":i32})
                }
              }
              n218 = Build Array(w449, w452, w451, w449) -> (w450:cluster{"X":i32, "Y":i32}[])
              n219 = call "IMAQ Overlay Multiple Lines 2"("Image"=w457, "Line End Points"=w450, "Color"=w455) -> ("Image Out"=w456:T1)  [unwired: 11 in, 1 out]
            }
          }
          n220 = call "IMAQ Overlay Line"("Color"=w408, "error in (no error)"=w436, "End Point"=w402, "Start Point"=w437, "Image"=w409) -> ("error out"=w426:errorcluster, "Image Out"=w407:T1)  [unwired: 5 in]
          n221 = call "IMAQ Convert Line to ROI"("error in (no error)"=w426, "Line"=w423) -> ("error out"=w418:errorcluster, "ROI Descriptor"=w417:T16)  [unwired: 7 in]
          n222 = call "IMAQ Edge Tool 3"("Image"=w407, "Edge Options"=w424, "Optimized Mode"=FALSE, "ROI Descriptor"=w417, "Process"=w428, "error in (no error)"=w418) -> ("Image (duplicate)"=w430:T1, "Edge Information"=w433:T17[], "Gradient Values"=w421:dbl[], "error out"=w419:errorcluster)  [unwired: 5 in, 1 out]
          n223 = call "IMAQ ROIProfile"("error in (no error)"=w419, "ROI Descriptor"=w417, "Image"=w407) -> ("error out"=w432:errorcluster, "ROI Graph"=w422:cluster{"x0":sgl, "dx":sgl, "Pixels Line":sgl[]})  [unwired: 1 in, 3 out]
          n224 = case shown="False" "單點" {
            tunnel: [w499 w510] -> w427
            tunnel: w433 -> [w501 w517]
            tunnel: [w504 w514] -> w420
            tunnel: w432 -> [w503 w512]
            tunnel: [w502 w511] -> w425
            tunnel: w430 -> [w498 w510]
            frame False {
              n225 = for {
                tunnel: w501 -> [w509] mode=indexing
                tunnel: [w508] -> w500 mode=indexing
                n226 = Unbundle By Name(w509) -> ("Location (Pixel)"=w508:cluster{"X":sgl, "Y":sgl})
              }
              n227 = Index Array(array=w501, index=0) -> (element=w505:T17)
              n228 = Unbundle By Name(w505) -> ("Location (Pixel)"=w504:cluster{"X":sgl, "Y":sgl})
              n229 = call "Overlay Points with User Specified Size.vi"("Color"=u32 16711680, "error in"=w503, "Points"=w500, "Image In"=w498) -> ("error out"=w502:errorcluster, "Image Out"=w499:T1)  [unwired: 6 in]
            }
            frame True {
              n230 = Index Array(array=w517, index=0) -> (element=w515:T17)
              n231 = Unbundle By Name(w515) -> ("Location (Pixel)"=w514:cluster{"X":sgl, "Y":sgl})
              n232 = Build Array(w514) -> (w513:cluster{"X":sgl, "Y":sgl}[])
              n233 = call "Overlay Points with User Specified Size.vi"("Color"=u32 16711680, "error in"=w512, "Points"=w513, "Image In"=w510) -> ("error out"=w511:errorcluster)  [unwired: 6 in, 1 out]
            }
          }
        }
        "Line Profile" <- w312
        n234 = flat-sequence {
          tunnel: w311 -> [w386]
          tunnel: [w386] -> w338
          tunnel: w338 -> [w388]
          frame #0 {
            n235 = property on="Gradient Information" class="WFChart (strict)"("History Data"=dbl[][] []) -> ()  [unwired: 2 in, 2 out]
          }
          frame #1 {
            n236 = Transpose 2D Array(2D array=w388) -> (transposed array=→"Gradient Information":dbl[][])
          }
        }
        n237 = for {
          tunnel: w310 -> [w392] mode=indexing
          shift-right: [w391] -> w340
          shift-left: cluster{"X":sgl, "Y":sgl}[] [] -> [w390]
          n238 = Unbundle By Name(w392) -> ("X"=w396:sgl, "Y"=w395:sgl)
          n239 = Multiply(x=w396, y=w395) -> (x*y=w394:sgl)
          n240 = Not Equal To 0?(x=w394) -> (x != 0?=w393:bool)
          n241 = case shown="True" w393 {
            tunnel: w392 -> [_ w400]
            tunnel: [w397 w399] -> w391
            tunnel: w390 -> [w397 w398]
            frame False {
            }
            frame True {
              n242 = Build Array (concatenate)(w398, w400) -> (w399:cluster{"X":sgl, "Y":sgl}[])
            }
          }
        }
        n243 = call "IMAQ Fit Line"("error in (no error)"=w308, "Pixel Radius"=sgl 10.0, "Points"=w340) -> ("error out"=w306:errorcluster, "Line Segment"=w305:T7)  [unwired: 3 in, 4 out]
        "Line Segment" <- w305
        n244 = Unbundle By Name(w305) -> ("Point 1"=w292:cluster{"X":sgl, "Y":sgl}, "Point 2"=w293:cluster{"X":sgl, "Y":sgl})
        n245 = Unbundle By Name(w292) -> ("X"=w302:sgl, "Y"=w300:sgl)
        n246 = Unbundle By Name(w293) -> ("X"=w301:sgl, "Y"=w299:sgl)
        n247 = call "IMAQ Overlay Line"("Color"=u32 16711680, "error in (no error)"=w306, "End Point"=w293, "Start Point"=w292, "Image"=w309) -> ("error out"=→"error out":errorcluster, "Image Out"=w304:T1)  [unwired: 5 in]
        n248 = Subtract(x=w302, y=w301) -> (x-y=w298:sgl)
        n249 = Subtract(x=w299, y=w300) -> (x-y=w297:sgl)
        n250 = Divide(x=w297, y=w298) -> (x/y=w296:sgl)
        n251 = Inverse Tangent(1:w296) -> (0:w295:sgl)
        n252 = expression code="(x/pi)*180.0" "radians to degrees"(w295) -> (→"degrees":sgl)
      }
    }
    "Image" <- w271
  }
